vi "Wait for Response.vi"(7 "Timeout (ms)":dbl, 8 "error in (no error)":errorcluster, 10 "Data cluster in":T1, 11 "VISA Refnum in":refnum<visa-resource-name>) -> (0 "error out":errorcluster, 1 "Pass?":bool, 2 "output cluster":T1, 3 "VISA Refnum out":refnum<visa-resource-name>)   [LabVIEW 2020]
uses:
  Data Cluster.ctl
panel:
  # "Send Data:"
  # "Receive Data:"
  # "Send Data:"
  # "Receive Data:"
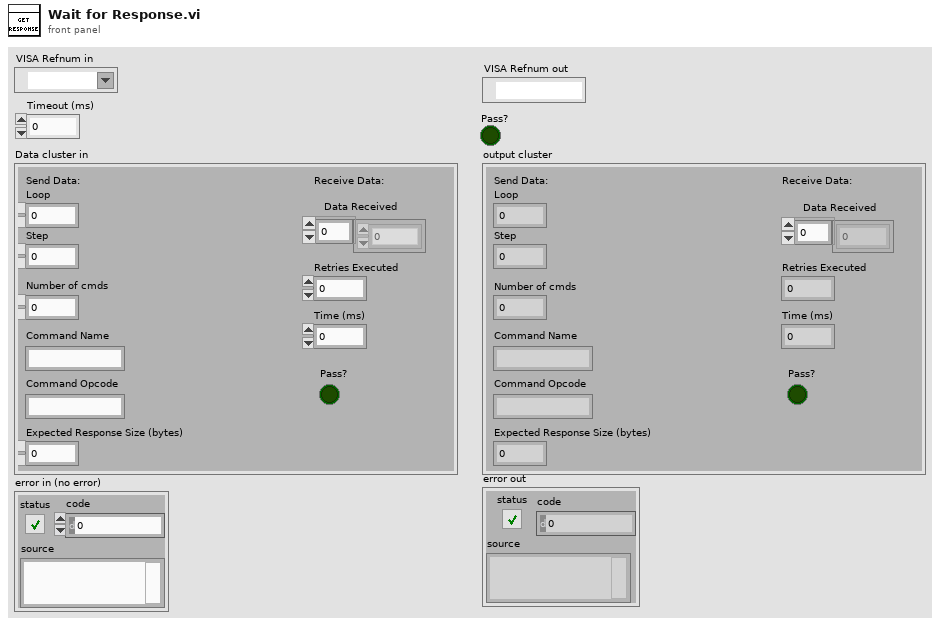
[diagram p1: front panel]
types:
  T1 = typedef "Data Cluster.ctl" = cluster{"Command Name":string, "Command Opcode ":string, "Step":dbl, "Loop":dbl, "Expected Response Size (bytes)":u16, "Number of cmds":dbl, "Data Received":u8[], "Retries Executed":u16, "Time (ms)":u16, "Pass?":bool}
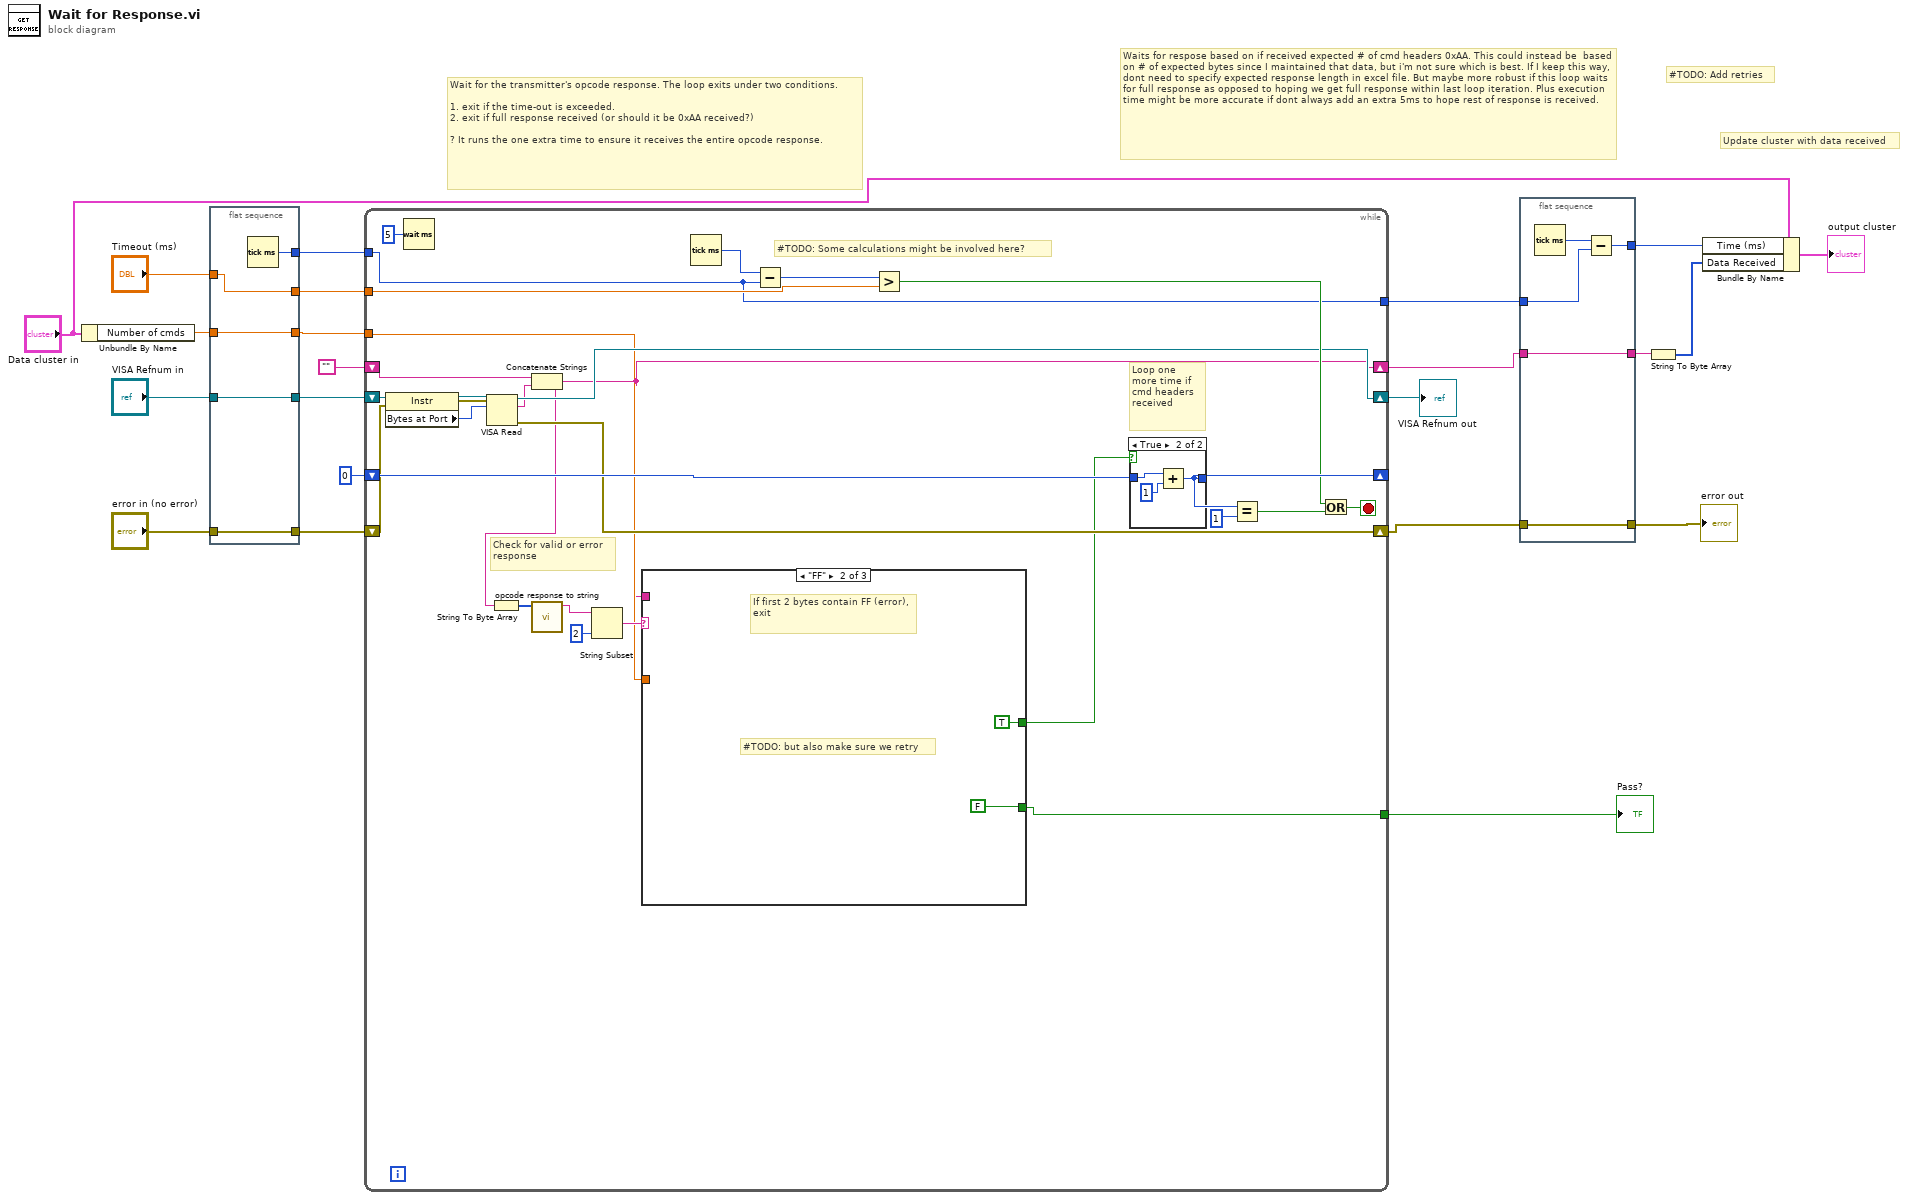
[diagram p0: block diagram]
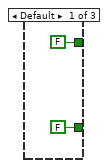
[diagram p2: hidden frame]
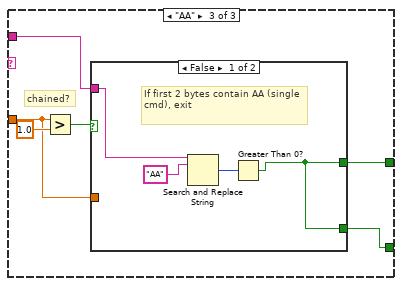
[diagram p3: hidden frame]
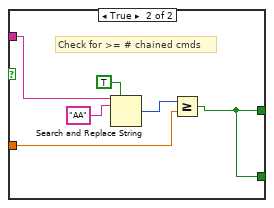
[diagram p4: hidden frame]
diagram:
  # "#TODO: Add retries"
  # "Update cluster with data received"
  # "Waits for respose based on if received expected # of cmd headers 0xAA. This could instead be  based on # of expected bytes since I maintained that data, but i'm not sure which is best. If I keep this way, dont need to specify expected response length in excel file. But maybe more robust if this loop waits for full response as opposed to hoping we get full response within last loop iteration. Plus execution time might be more accurate if dont always add an extra 5ms to hope rest of response is received."
  # "Wait for the transmitter's opcode response. The loop exits under two conditions. \n\n1. exit if the time-out is exceeded. \n2. exit if full response received (or should it be 0xAA received?)\n\n? It runs the one extra time to ensure it receives the entire opcode response."
  n1 = Unbundle By Name("Data cluster in") -> ("Number of cmds"=w4:dbl)
  n2 = flat-sequence {
    tunnel: [w27] -> w16
    tunnel: "VISA Refnum in" -> [w26]
    tunnel: [w26] -> w20
    tunnel: "error in (no error)" -> [w25]
    tunnel: [w25] -> w18
    tunnel: "Timeout (ms)" -> [w24]
    tunnel: [w24] -> w14
    tunnel: w4 -> [w23]
    tunnel: [w23] -> w3
    frame #0 {
      n3 = Tick Count (ms)() -> (millisecond timer value=w27:u32)
    }
  }
  n4 = while {
    tunnel: w3 -> [w33]
    shift-right: [w47] -> _
    shift-left: 0 -> [w51]
    shift-right: [w40] -> w17
    shift-left: w20 -> [w46]
    shift-right: [w39] -> w13
    shift-left: w18 -> [w45]
    tunnel: w16 -> [w38]
    tunnel: w14 -> [w42]
    tunnel: [w38] -> w11
    tunnel: [w32] -> w2
    shift-right: [w31] -> w7
    shift-left: "" -> [w28]
    stop <- w52 stop-if-true
    # "Check for valid or error response"
    # "#TODO: Some calculations might be involved here?"
    # "Loop one more time if cmd headers received"
    n5 = property class="Instr"(reference=w46, error in=w45) -> (reference out=w54:refnum<visa-resource-name>, error out=w53:errorcluster, "Bytes at Port"=w55:u32)
    n6 = Wait (ms)(milliseconds to wait=u32 5) -> ()  [unwired: 1 out]
    n7 = VISA Read(VISA resource name=w54, byte count=w55, error in (no error)=w53) -> (VISA resource name out=w40:refnum<visa-resource-name>, read buffer=w37:string, error out=w39:errorcluster)  [unwired: 1 out]
    n8 = Concatenate Strings(w28, w37) -> (w31:string)
    n9 = String To Byte Array(string=w31) -> (unsigned byte array=w30:u8[])
    n10 = call "opcode response to string.vi"("Data Received"=w30) -> ("Response String"=w29:string)  [unwired: 10 in]
    n11 = String Subset(string=w29, length (rest)=2 ("length (rest)")) -> (substring=w34:string)  [unwired: 1 in]
    n12 = case shown="\"FF\"" w34 {
      tunnel: w33 -> [_ _ w62]
      tunnel: [FALSE TRUE w63] -> w35
      tunnel: w31 -> [_ _ w61]
      tunnel: [FALSE FALSE w60] -> w32
      frame Default {
      }
      frame "FF" {
        # "#TODO: but also make sure we retry"
        # "If first 2 bytes contain FF (error), exit"
      }
      frame "AA" {
        # "chained?"
        n13 = Greater?(x=w62, y=1.0) -> (0:w64:bool)
        n14 = case shown="False" w64 {
          tunnel: [w66 w70] -> w63
          tunnel: w62 -> [_ w72]
          tunnel: w61 -> [w68 w71]
          tunnel: [w66 w70] -> w60
          frame False {
            # "If first 2 bytes contain AA (single cmd), exit"
            n15 = Search and Replace String(input string=w68, search string="AA") -> (number of replacements=w67:i32)  [unwired: 6 in, 3 out]
            n16 = Greater Than 0?(x=w67) -> (x > 0?=w66:bool)
          }
          frame True {
            # "Check for >= # chained cmds"
            n17 = Search and Replace String(replace all?=TRUE ("replace all? (F)"), input string=w71, search string="AA") -> (number of replacements=w73:i32)  [unwired: 5 in, 3 out]
            n18 = Greater Or Equal?(x=w73, y=w72) -> (x >= y?=w70:bool)
          }
        }
      }
    }
    n19 = Tick Count (ms)() -> (millisecond timer value=w44:u32)
    n20 = Subtract(x=w44, y=w38) -> (x-y=w43:u32)
    n21 = Greater?(x=w43, y=w42) -> (0:w41:bool)
    n22 = case shown="True" w35 {
      tunnel: w51 -> [w76 w78]
      tunnel: [w76 w79] -> w47
      frame False {
      }
      frame True {
        n23 = Add(x=w78, y=1) -> (x+y=w79:i32)
      }
    }
    n24 = Equal?(x=w47, y=1) -> (x = y?=w48:bool)
    n25 = Or(x=w41, y=w48) -> (x .or. y?=w52:bool)
  }
  "VISA Refnum out" <- w17
  "Pass?" <- w2
  n26 = flat-sequence {
    tunnel: w11 -> [w84]
    tunnel: [w83] -> w10
    tunnel: w13 -> [w81]
    tunnel: [w81] -> w12
    tunnel: w7 -> [w80]
    tunnel: [w80] -> w6
    frame #0 {
      n27 = Tick Count (ms)() -> (millisecond timer value=w82:u32)
      n28 = Subtract(x=w82, y=w84) -> (x-y=w83:u32)
    }
  }
  n29 = String To Byte Array(string=w6) -> (unsigned byte array=w9:u8[])
  n30 = Bundle By Name(cluster="Data cluster in", "Time (ms)"=w10, "Data Received"=w9) -> (→"output cluster":T1)
  "error out" <- w12
